vi "OnInit.vi"(8 "error in (no error)":errorcluster, 11 "Game in":refnum<class "Game.lvclass">) -> (0 "error out":errorcluster, 3 "Game out":refnum<class "Game.lvclass">)   [LabVIEW 2019, in "RT_Game.lvlib" / "Game.lvclass"]
uses:
  Game.lvclass
  Menu/States.ctl
  Game.lvclass/Game.ctl
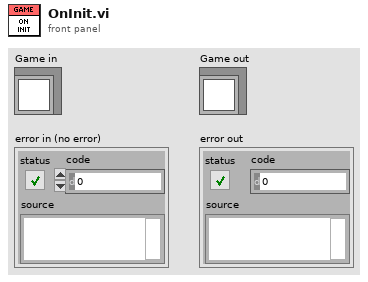
[diagram p1: front panel]
types:
  T1 = typedef "RT_Game.lvlib/Game.lvclass/States.ctl" = enum16{"Init", "Restart", "Menu", "Game", "Resume", "ToggleSingleplayer", "LoadNextGame", "ExitToMenu", "NewHighscore", "GameOver", "SlideOut"}
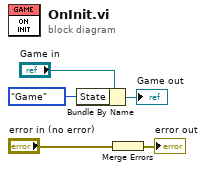
[diagram p0: block diagram]
diagram:
  n1 = Bundle By Name(cluster="Game in", "State"=States."Game") -> (→"Game out":refnum<class "Game.lvclass">)
  n2 = Merge Errors("error in (no error)") -> (→"error out":errorcluster)
